vi "Push All Ctrls.vi"(8 "error in":errorcluster, 11 "OpticalPrime Ctrls For Saving":T1={"Time Stamp"={"date string"="", "time string"=""}, "Exp Params"={"Experiment Type"="Time Series", "Experiment Name"="Experiment_1", "ExpPath"=path "D:/Data", "Save As"="TIFF", "TSFrames"=1000, "TSfps"=1.0, "Streaming"=TRUE, "tdms ref"=refnum, "frame #"=0, "Full Path"=path "", "PeakOnQueue"=FALSE}, "Ventus Controls"={"Ventus Power"=0.0, "Open Serial"=FALSE, "VISA Refnum"=""}, "Camera Controls"={"Exposure Time (ms)"=27, "cam0 Session"="", "Camera ROI"={"Width"=0, "Height"=0, "Offset X"=0, "Offset Y"=0}, "Command"=""}, "Spot Params"=[], "SLM Parameters"={"Width"=0.0, "Height"=0.0, "Board ID"=0, "Centre Y"=0.0, "Centre X"=0.0}} {"Spot Params"."Z" format="%_4g"; "Spot Params"."Y" format="%_4g"; "Spot Params"."X" format="%_4g"; "Spot Params"."Phase" format="%_4g"; "Spot Params"."Intensity" format="%_4g"; "Camera Controls"."Camera ROI"."Offset Y" max=2046 step=2; "Camera Controls"."Camera ROI"."Offset X" max=2044 step=4; "Camera Controls"."Camera ROI"."Height" min=2 max=2048 step=2; "Camera Controls"."Camera ROI"."Width" min=4 max=2048 step=4; "Camera Controls"."Exposure Time (ms)" min=27 max=500 step=1 scale=27.0..500.0; "SLM Parameters"."Centre X" format="%.3g"; "SLM Parameters"."Centre Y" format="%.3g"; "Ventus Controls"."Ventus Power" min=0.0 max=100.0 step=0.1 scale=0.0..100.0; "Exp Params"."TSFrames" min=1 step=1; "Exp Params"."TSfps" min=0.001 max=90.0 step=0.001 format="%_4g"}) -> (0 "error out":errorcluster, 3 "OpticalPrime Ctrls For Saving out":T1={"Time Stamp"={"date string"="", "time string"=""}, "Exp Params"={"Experiment Type"="Time Series", "Experiment Name"="Experiment_1", "ExpPath"=path "D:/Data", "Save As"="TIFF", "TSFrames"=1000, "TSfps"=1.0, "Streaming"=TRUE, "tdms ref"=refnum, "frame #"=0, "Full Path"=path "", "PeakOnQueue"=FALSE}, "Ventus Controls"={"Ventus Power"=0.0, "Open Serial"=FALSE, "VISA Refnum"=""}, "Camera Controls"={"Exposure Time (ms)"=27, "cam0 Session"="", "Camera ROI"={"Width"=0, "Height"=0, "Offset X"=0, "Offset Y"=0}, "Command"=""}, "Spot Params"=[], "SLM Parameters"={"Width"=0.0, "Height"=0.0, "Board ID"=0, "Centre Y"=0.0, "Centre X"=0.0}} {"Spot Params"."Z" format="%_4g"; "Spot Params"."Y" format="%_4g"; "Spot Params"."X" format="%_4g"; "Spot Params"."Phase" format="%_4g"; "Spot Params"."Intensity" format="%_4g"; "Camera Controls"."Camera ROI"."Offset Y" max=2046 step=2; "Camera Controls"."Camera ROI"."Offset X" max=2044 step=4; "Camera Controls"."Camera ROI"."Height" min=2 max=2048 step=2; "Camera Controls"."Camera ROI"."Width" min=4 max=2048 step=4; "Camera Controls"."Exposure Time (ms)" min=27 max=500 step=1 scale=27.0..500.0; "SLM Parameters"."Centre X" format="%.3g"; "SLM Parameters"."Centre Y" format="%.3g"; "Ventus Controls"."Ventus Power" min=0.0 max=100.0 step=0.1 scale=0.0..100.0; "Exp Params"."TSFrames" min=1 step=1; "Exp Params"."TSfps" min=0.001 max=90.0 step=0.001 format="%_4g"})   [LabVIEW 2020]
uses:
  _controls/OpticalPrime Ctrls For Saving.ctl
  _controls/Exp Params.ctl
  _controls/Ventus Control.ctl
  _controls/xiCam.ctl
  <vilib>/userDefined/High Color/IMAQdx.ctl
  _controls/Spot Params.ctl
  _controls/PCIe SLM params.ctl
  _globals/OpticalPrime Controls.vi
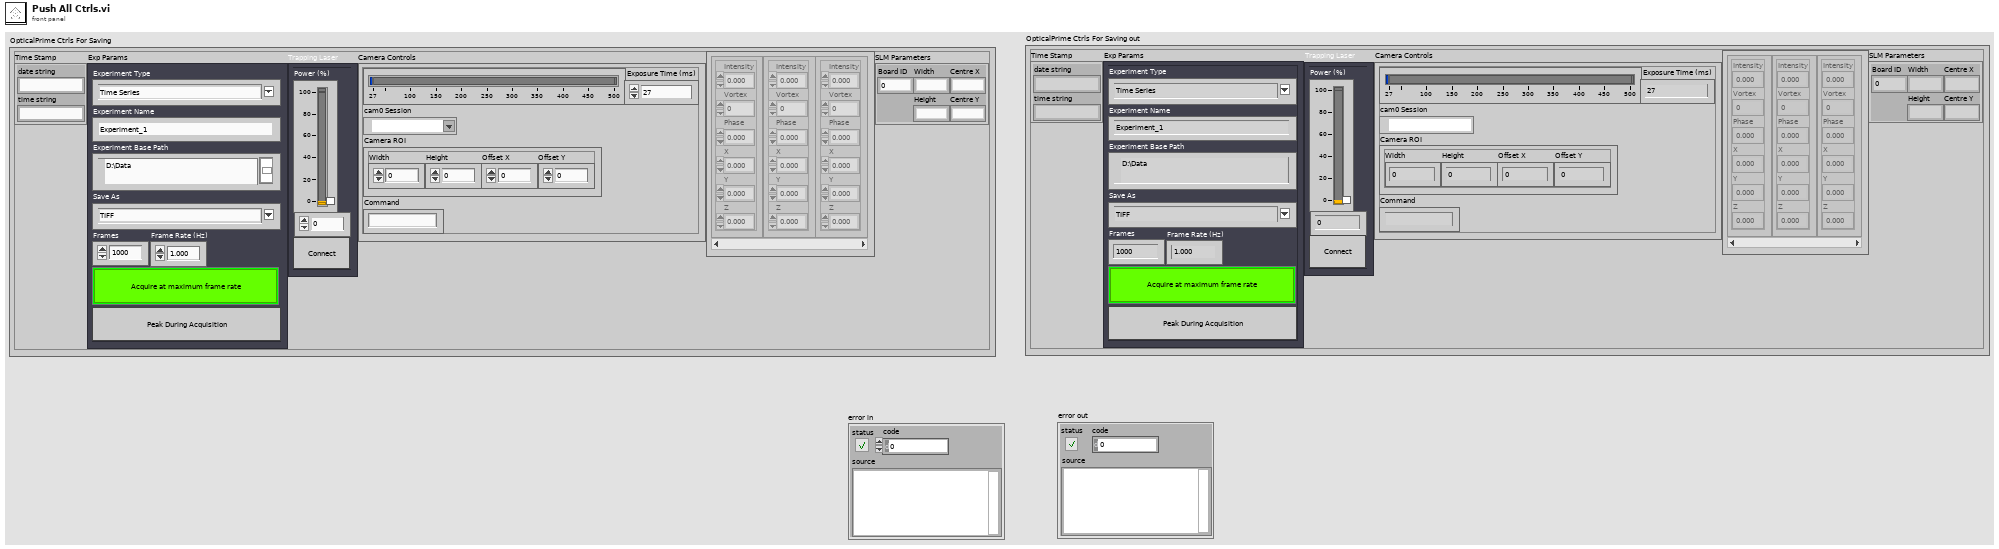
[diagram p1: front panel]
types:
  T1 = typedef "OpticalPrime Ctrls For Saving.ctl" = cluster{"Time Stamp":cluster{"date string":string, "time string":string}, "Exp Params":T2, "Ventus Controls":T3, "Camera Controls":T4, "Spot Params":T6, "SLM Parameters":T7}
  T2 = typedef "Exp Params.ctl" = cluster{"Experiment Type":string, "Experiment Name":string, "ExpPath":path, "Save As":string, "TSFrames":i32, "TSfps":dbl, "Streaming":bool, "tdms ref":refnum<k34>, "frame #":i64, "Full Path":path, "PeakOnQueue":bool}
  T3 = typedef "Ventus Control.ctl" = cluster{"Ventus Power":dbl, "Open Serial":bool, "VISA Refnum":refnum<visa-resource-name>}
  T4 = typedef "xiCam.ctl" = cluster{"Exposure Time (ms)":u32, "cam0 Session":T5, "Camera ROI":cluster{"Width":u32, "Height":u32, "Offset X":u32, "Offset Y":u32}, "Command":string}
  T5 = typedef "IMAQdx.ctl" = refnum<k21>
  T6 = typedef "Spot Params.ctl" = cluster{"Intensity":dbl, "Vortex":dbl, "Phase":dbl, "X":dbl, "Y":dbl, "Z":dbl}[]
  T7 = typedef "PCIe SLM params.ctl" = cluster{"Width":dbl, "Height":dbl, "Board ID":i32, "Centre Y":dbl, "Centre X":dbl}
  T8 = typedef "OpticalPrime Ctrl Refs.ctl" = cluster{"Exp Params":refnum<vi>, "Ventus Controls":refnum<vi>, "SLM Parameters":refnum<vi>, "Spot Params":refnum<vi>, "Camera Controls":refnum<vi>}
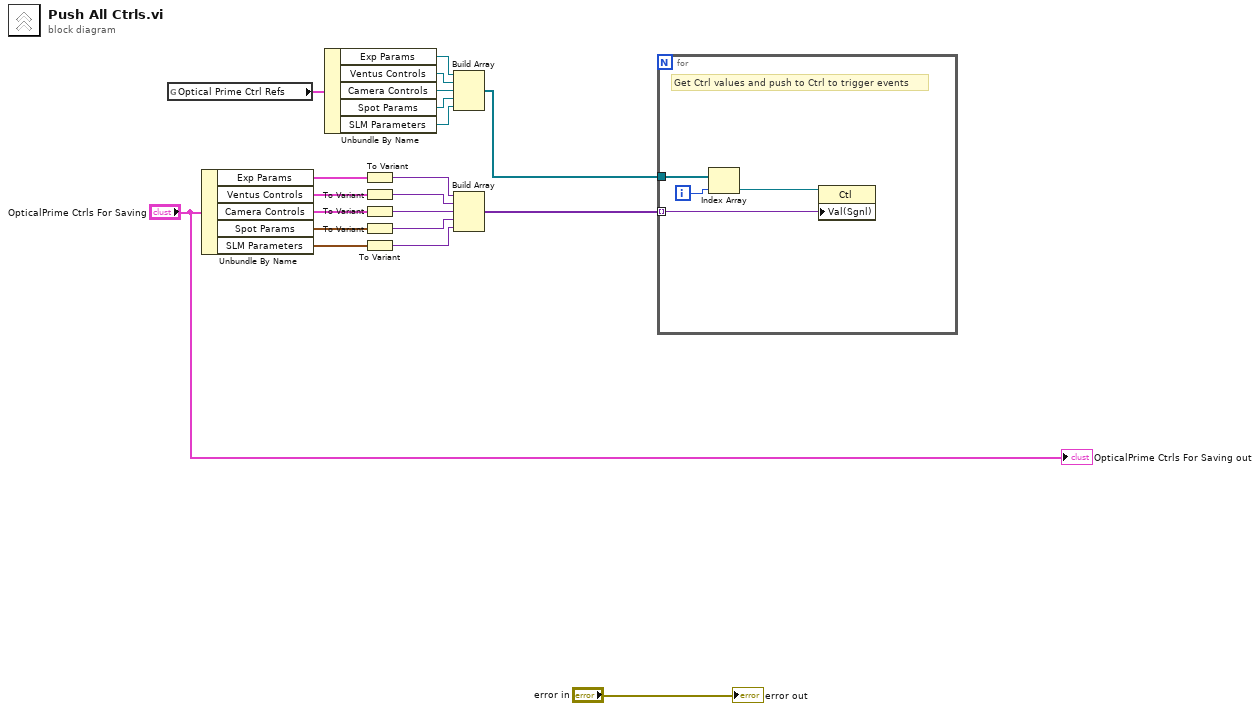
[diagram p0: block diagram]
diagram:
  n1 = global read "OpticalPrime Controls.vi" "Optical Prime Ctrl Refs"() -> (w11:T8)
  n2 = Unbundle By Name("OpticalPrime Ctrls For Saving") -> ("Exp Params"=w19:T2, "Ventus Controls"=w18:T3, "Camera Controls"=w4:T4, "Spot Params"=w17:T6, "SLM Parameters"=w16:T7)
  n3 = Unbundle By Name(w11) -> ("Exp Params"=w10:refnum<vi>, "Ventus Controls"=w9:refnum<vi>, "Camera Controls"=w1:refnum<vi>, "Spot Params"=w8:refnum<vi>, "SLM Parameters"=w7:refnum<vi>)
  n4 = To Variant(anything=w19) -> (Variant=w15:variant)
  n5 = To Variant(anything=w18) -> (Variant=w14:variant)
  n6 = To Variant(anything=w4) -> (Variant=w2:variant)
  n7 = To Variant(anything=w17) -> (Variant=w3:variant)
  n8 = To Variant(anything=w16) -> (Variant=w13:variant)
  n9 = Build Array(w10, w9, w1, w8, w7) -> (w6:refnum<vi>[])
  n10 = Build Array(w15, w14, w2, w3, w13) -> (w12:variant[])
  n11 = for {
    tunnel: w12 -> [w22] mode=indexing
    tunnel: w6 -> [w24]
    i -> [w23]
    # "Get Ctrl values and push to Ctrl to trigger events"
    n12 = Index Array(array=w24, index=w23) -> (element=w21:refnum<vi>)
    n13 = property class="Ctl"(reference=w21, "Val(Sgnl)"=w22) -> ()  [unwired: 1 in, 2 out]
  }
  "error out" <- "error in"
  "OpticalPrime Ctrls For Saving out" <- "OpticalPrime Ctrls For Saving"
